vi "test1-testModuleExitEventAPI.vi"(8 "error in (no error)":errorcluster, 11 "TestCase in":refnum<class "testcase-CSMNonCSMCallerSupportAPI.lvclass">) -> (0 "error out":errorcluster, 3 "TestCase out":refnum<class "testcase-CSMNonCSMCallerSupportAPI.lvclass">)   [LabVIEW 2017, in "testcase-CSMNonCSMCallerSupportAPI.lvclass"]
uses:
  testcase-CSMNonCSMCallerSupportAPI.lvclass
  src/user.lib/_NEVSTOP/Communicable State Machine(CSM)/_Support/Typedef/_CSM_List Module Scope.ctl
  InternalCluster.ctl
  State_Cluster.ctl
  GlobalVariable_CSMModeData.vi
  <vilib>/addons/_JKI Toolkits/VI Tester/TestCase.llb/TestCase.lvclass
  src/user.lib/_NEVSTOP/Communicable State Machine(CSM)/Communicable State Machine.lvlib
  C:/Program Files (x86)/National Instruments/LabVIEW 2017/vi.lib/addons/_JKI Toolkits/VI Tester/TestCase.llb/TestCase.lvclass
panel:
  out "error out 2":errorcluster
  out "LoopCount":i32
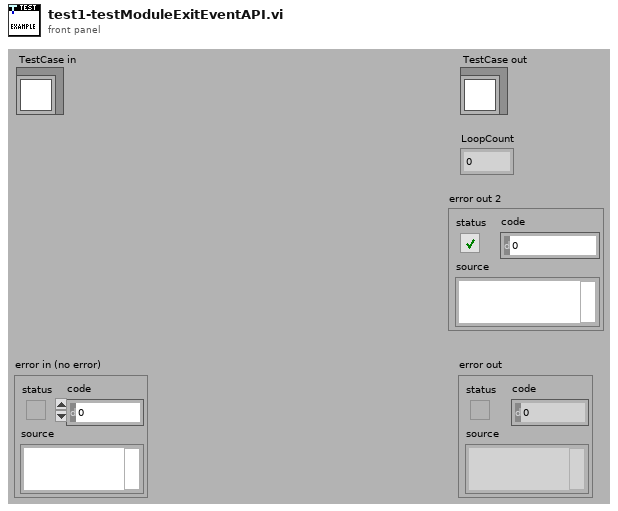
[diagram p1: front panel]
types:
  T1 = typedef "testcase-CSMNonCSMCallerSupportAPI.lvclass/InternalCluster.ctl" = cluster{"Mode":enum16{"Invalid", "Others", "WorkerAgent or Chain"}, "#Nodes":u32}
  T2 = typedef "Communicable State Machine.lvlib/_CSM_List Module Scope.ctl" = enum16{"Normal", "System Only", "All"}
  T3 = typedef "testcase-CSMNonCSMCallerSupportAPI.lvclass/State_Cluster.ctl" = enum16{"Idle", "Initialize", "PreExit", "Exit"}
  T4 = enum16{"Invalid", "Others", "WorkerAgent or Chain"}
  T5 = typedef "Communicable State Machine.lvlib/_CSM_MODE.ctl" = enum16{"Not Exist", "Stand Alone", "CSM", "Worker", "Worker Agent", "Chain Node", "Chain"}
  T6 = cluster{"Module Exit event occured":bool, "Exit until all nodes exited":bool}
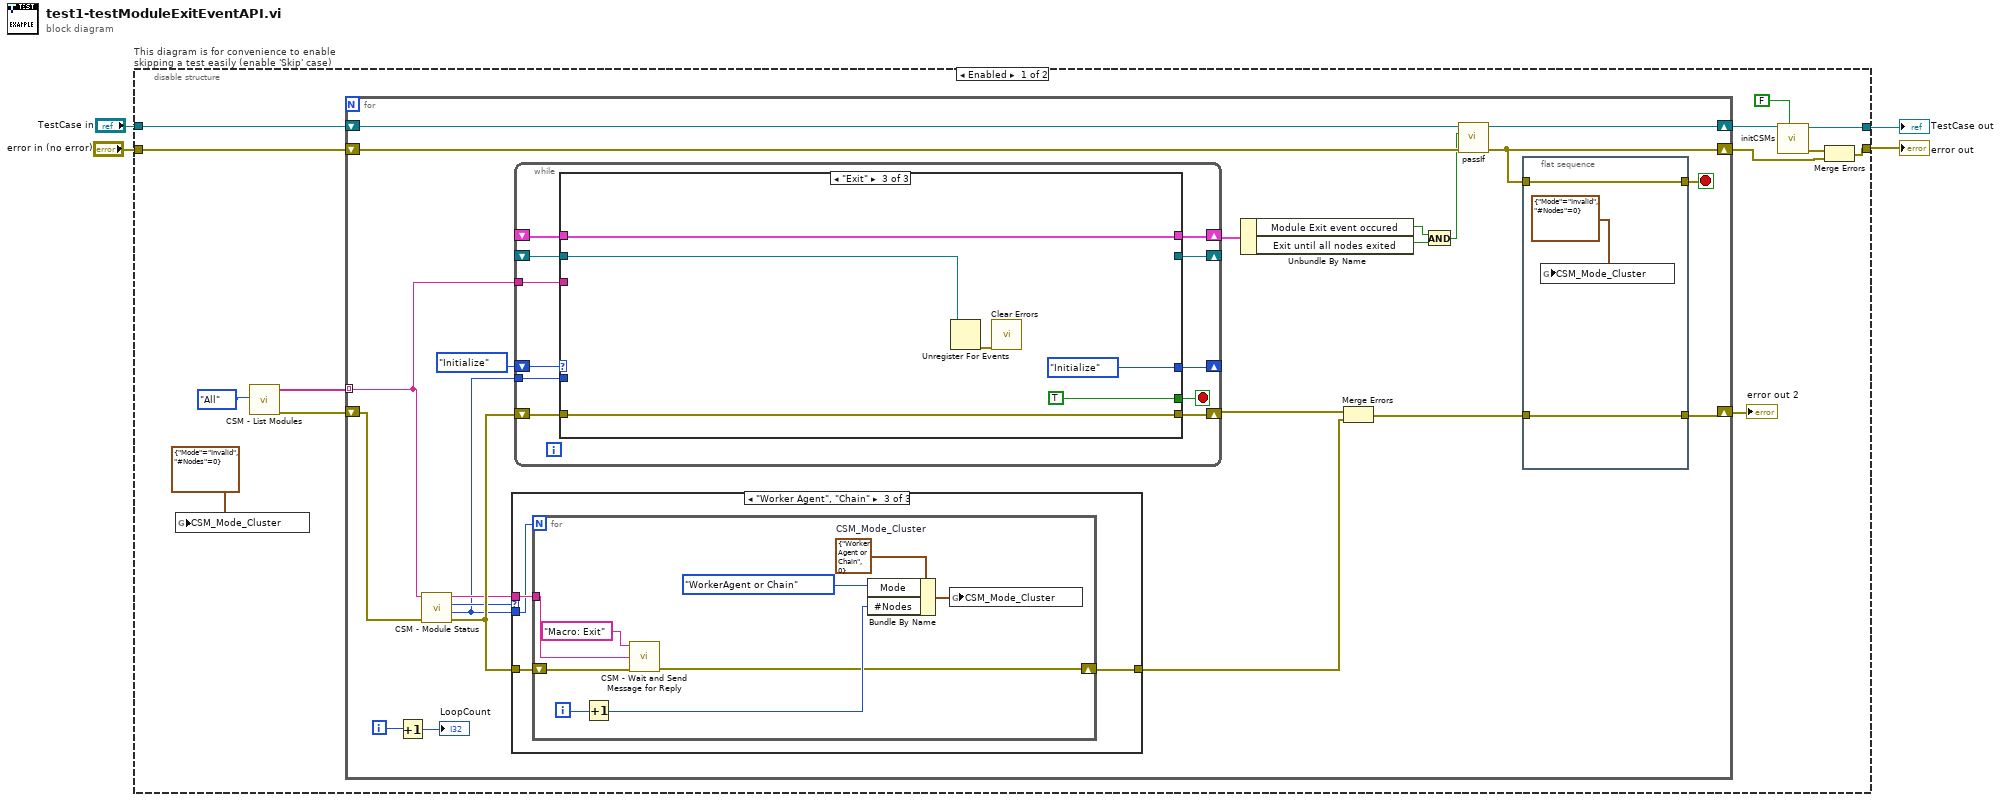
[diagram p0: block diagram]
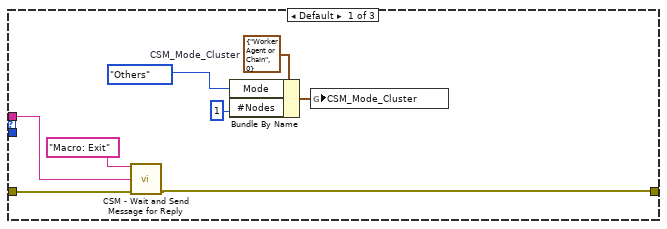
[diagram p2: hidden frame]
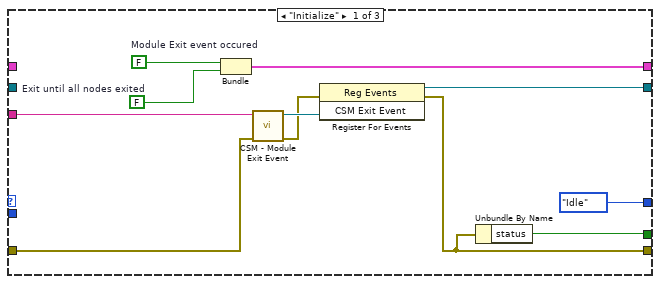
[diagram p4: hidden frame]
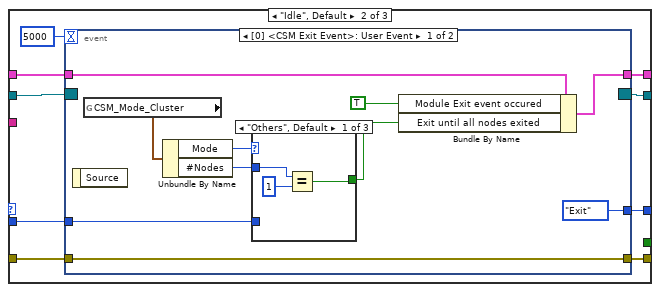
[diagram p5: hidden frame]
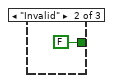
[diagram p6: hidden frame]
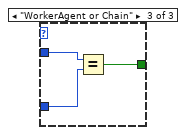
[diagram p7: hidden frame]
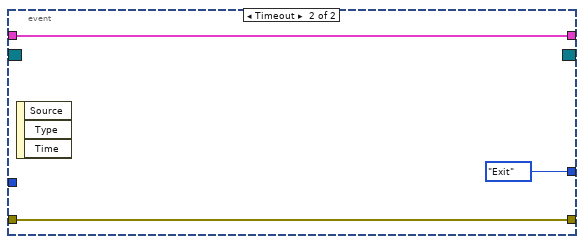
[diagram p8: hidden frame]
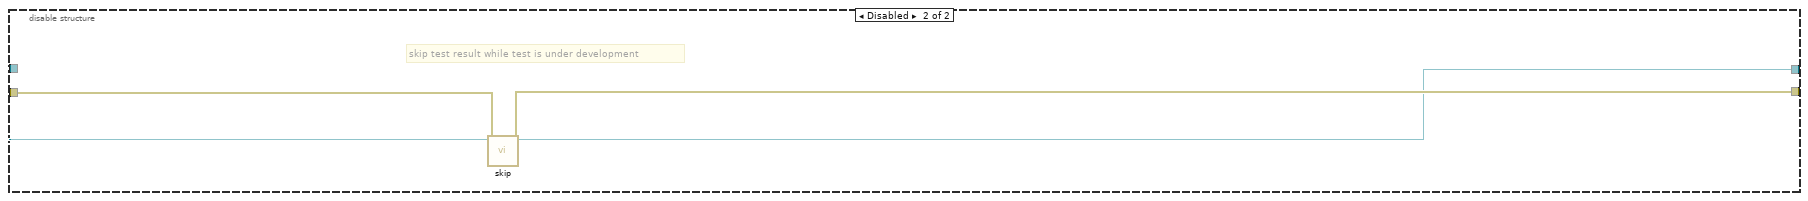
[diagram p9: hidden frame]
diagram:
  n1 = disable-structure "This diagram is for convenience to enable skipping a test easily (enable 'Skip' case)" shown="Enabled" {
    disable-tunnel: "TestCase in" -> [w15 w125]
    disable-tunnel: [w11 w123] -> w1
    disable-tunnel: [w8 w124] -> w3
    disable-tunnel: "error in (no error)" -> [w14 w122]
    frame Enabled {
      n2 = global write "GlobalVariable_CSMModeData.vi" "CSM_Mode_Cluster"(T1 {"Mode"=enum."Invalid", "#Nodes"=0} ("CSM_Mode_Cluster")) -> ()
      n3 = call "CSM - List Modules.vi"("Scope (Normal)"=_CSM_List_Module_Scope."All") -> ("error out"=w16:errorcluster, "Module Names"=w5:string[])  [unwired: 9 in]
      n4 = for {
        shift-right: [w18] -> w7
        shift-left: w16 -> [w29]
        shift-right: [w21] -> w12
        shift-left: w15 -> [w36]
        shift-right: [w20] -> w9
        shift-left: w14 -> [w35]
        tunnel: w5 -> [w22] mode=indexing
        i -> [w38]
        stop <- w23 stop-if-true
        n5 = Increment(x=w38) -> (x+1=→"LoopCount":i32)
        n6 = call "CSM - Module Status.vi"("Error In"=w29, "CSM Name"=w22) -> ("error out"=w27:errorcluster, "#Nodes"=w24:i32, "Mode"=w26:T5, "CSM Name (Dup)"=w25:string)  [unwired: 5 in, 1 out]
        n7 = case shown="\"Worker Agent\", \"Chain\"" w26 {
          tunnel: w27 -> [w50 w51 w55]
          tunnel: w24 -> [_ _ w53]
          tunnel: w25 -> [w48 _ w54]
          tunnel: [w43 w51 w52] -> w28
          frame Default {
            w47 = T1 {"Mode"=enum."WorkerAgent or Chain", "#Nodes"=0}  # CSM_Mode_Cluster
            n8 = call "CSM - Wait and Send Message for Reply.vi"("State"="Macro: Exit", "Target Module"=w48, "Error In (No Error)"=w50) -> ("error out"=w43:errorcluster)  [unwired: 9 in, 3 out]
            n9 = Bundle By Name(cluster=w47, "Mode"=T4."Others", "#Nodes"=u32 1) -> (w46:T1)
            n10 = global write "GlobalVariable_CSMModeData.vi" "CSM_Mode_Cluster"(w46) -> ()
          }
          frame "Not Exist" {
          }
          frame "Worker Agent", "Chain" {
            n11 = for {
              N: w53 -> [_]
              shift-right: [w56] -> w52
              shift-left: w55 -> [w64]
              tunnel: w54 -> [w61]
              i -> [w62]
              w60 = T1 {"Mode"=enum."WorkerAgent or Chain", "#Nodes"=0}  # CSM_Mode_Cluster
              n12 = Increment(x=w62) -> (x+1=w58:i32)
              n13 = call "CSM - Wait and Send Message for Reply.vi"("State"="Macro: Exit", "Target Module"=w61, "Error In (No Error)"=w64) -> ("error out"=w56:errorcluster)  [unwired: 9 in, 3 out]
              n14 = Bundle By Name(cluster=w60, "Mode"=T4."WorkerAgent or Chain", "#Nodes"=w58) -> (w59:T1)
              n15 = global write "GlobalVariable_CSMModeData.vi" "CSM_Mode_Cluster"(w59) -> ()
            }
          }
        }
        n16 = while {
          shift-right: [w70] -> _
          shift-left: State_Cluster."Initialize" -> [w68]
          shift-right: [w74] -> _
          shift-left: _ -> [w73]
          shift-right: [w72] -> w33
          shift-left: _ -> [w69]
          shift-right: [w71] -> w34
          shift-left: w27 -> [w66]
          tunnel: w24 -> [w67]
          tunnel: w22 -> [w65]
          stop <- w75 stop-if-true
          n17 = case shown="\"Exit\"" w68 {
            tunnel: [w83 _ TRUE] -> w75
            tunnel: [w85 w94 _] -> w74
            tunnel: w73 -> [_ w95 w121]
            tunnel: [w78 w92 w119] -> w72
            tunnel: w69 -> [_ w93 w119]
            tunnel: w66 -> [w84 w89 w117]
            tunnel: [w81 w88 w117] -> w71
            tunnel: [State_Cluster."Idle" w90 State_Cluster."Initialize"] -> w70
            tunnel: w67 -> [_ w87 _]
            tunnel: w65 -> [w76 _ _]
            frame "Initialize" {
              w77 = FALSE  # Exit until all nodes exited
              w79 = FALSE  # Module Exit event occured
              n18 = Bundle("Module Exit event occured"=w79, "Exit until all nodes exited"=w77) -> (w78:T6)  [unwired: 1 in]
              n19 = call "CSM - Module Exit Event.vi"("Error In"=w84, "Name (\"\" to Use UUID) In"=w76) -> ("error out"=w82:errorcluster, "CSM Exit Event"=w86:refnum<user-event>)  [unwired: 7 in, 1 out]
              n20 = register-events(error in=w82, w86) -> (reference out=w85:refnum<event-registration>, error out=w81:errorcluster)  [unwired: 1 in]
              n21 = Unbundle By Name(w81) -> ("status"=w83:bool)
            }
            frame "Idle", Default {
              n22 = event shown="[0] <CSM Exit Event>: User Event" {
                selector: w95 -> [_ _]
                dyn-events: [_ _] -> w94
                timeout: 5000 -> [_ _]
                tunnel: [State_Cluster."Exit" State_Cluster."Exit"] -> w90
                tunnel: w93 -> [w104 w115]
                tunnel: [w97 w115] -> w92
                tunnel: w89 -> [w102 w113]
                tunnel: [w102 w113] -> w88
                tunnel: w87 -> [w98 _]
                event User Event {
                  n23 = event-data() -> ()  [unwired: 1 in, 1 out]
                  n24 = global read "GlobalVariable_CSMModeData.vi" "CSM_Mode_Cluster"() -> (w101:T1)
                  n25 = Unbundle By Name(w101) -> ("Mode"=w100:T4, "#Nodes"=w99:u32)
                  n26 = case shown="\"Others\", Default" w100 {
                    tunnel: [w106 FALSE w110] -> w96
                    tunnel: w99 -> [w108 _ w112]
                    tunnel: w98 -> [_ _ w111]
                    frame "Others", Default {
                      n27 = Equal?(x=w108, y=u32 1) -> (x = y?=w106:bool)
                    }
                    frame "Invalid" {
                    }
                    frame "WorkerAgent or Chain" {
                      n28 = Equal?(x=w112, y=w111) -> (x = y?=w110:bool)
                    }
                  }
                  n29 = Bundle By Name(cluster=w104, "Module Exit event occured"=TRUE, "Exit until all nodes exited"=w96) -> (w97:T6)
                }
                event Timeout {
                  n30 = event-data() -> ()  [unwired: 1 in, 3 out]
                }
              }
            }
            frame "Exit" {
              n31 = Unregister For Events(event registration refnum=w121) -> (error out=w120:errorcluster)  [unwired: 1 in]
              n32 = call <vilib>:"Clear Errors.vi"("error in (no error)"=w120) -> ()  [unwired: 5 in, 2 out]
            }
          }
        }
        n33 = Unbundle By Name(w33) -> ("Module Exit event occured"=w32:bool, "Exit until all nodes exited"=w31:bool)
        n34 = Merge Errors(w34, w28) -> (w19:errorcluster)
        n35 = And(x=w32, y=w31) -> (x .and. y?=w30:bool)
        n36 = call-dynamic "passIf.vi"("error in (no error)"=w35, "pass"=w30, "TestCase in"=w36) -> ("error out"=w20:errorcluster, "TestCase out"=w21:refnum<class "testcase-CSMNonCSMCallerSupportAPI.lvclass">)  [unwired: 7 in]
        n37 = flat-sequence {
          tunnel: w20 -> [w41]
          tunnel: [w41] -> w23
          tunnel: w19 -> [w40]
          tunnel: [w40] -> w18
          frame #0 {
            n38 = global write "GlobalVariable_CSMModeData.vi" "CSM_Mode_Cluster"(T1 {"Mode"=enum."Invalid", "#Nodes"=0} ("CSM_Mode_Cluster")) -> ()
          }
        }
      }
      "error out 2" <- w7
      n39 = call "initCSMs.vi"("Enable building lvlibp?"=FALSE, "TestCase in"=w12) -> ("error out"=w10:errorcluster, "TestCase out"=w11:refnum<class "testcase-CSMNonCSMCallerSupportAPI.lvclass">)  [unwired: 8 in]
      n40 = Merge Errors(w10, w9) -> (w8:errorcluster)
    }
    frame Disabled {
      # "skip test result while test is under development"
      n41 = call <vilib>:"skip.vi"("error in (no error)"=w122, "TestCase in"=w125) -> ("error out"=w124:errorcluster, "TestCase out"=w123:refnum<class "testcase-CSMNonCSMCallerSupportAPI.lvclass">)  [unwired: 8 in]
    }
  }
  "error out" <- w3
  "TestCase out" <- w1
